vi "Get Error Details (Default).vi"(11 "error":errorcluster) -> (1 "Message":string, 2 "Stack Trace":string, 3 "Type":string)   [LabVIEW 2013, in "JUnit Conversion.lvlib"]
uses:
  JUnit Conversion.lvlib
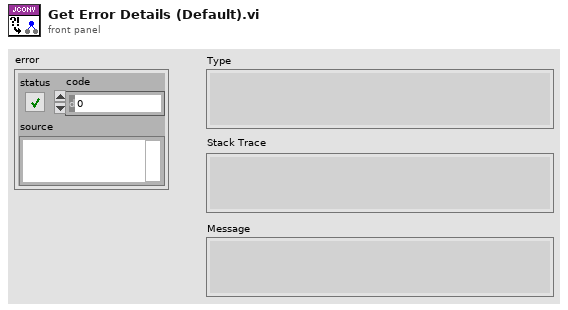
[diagram p1: front panel]
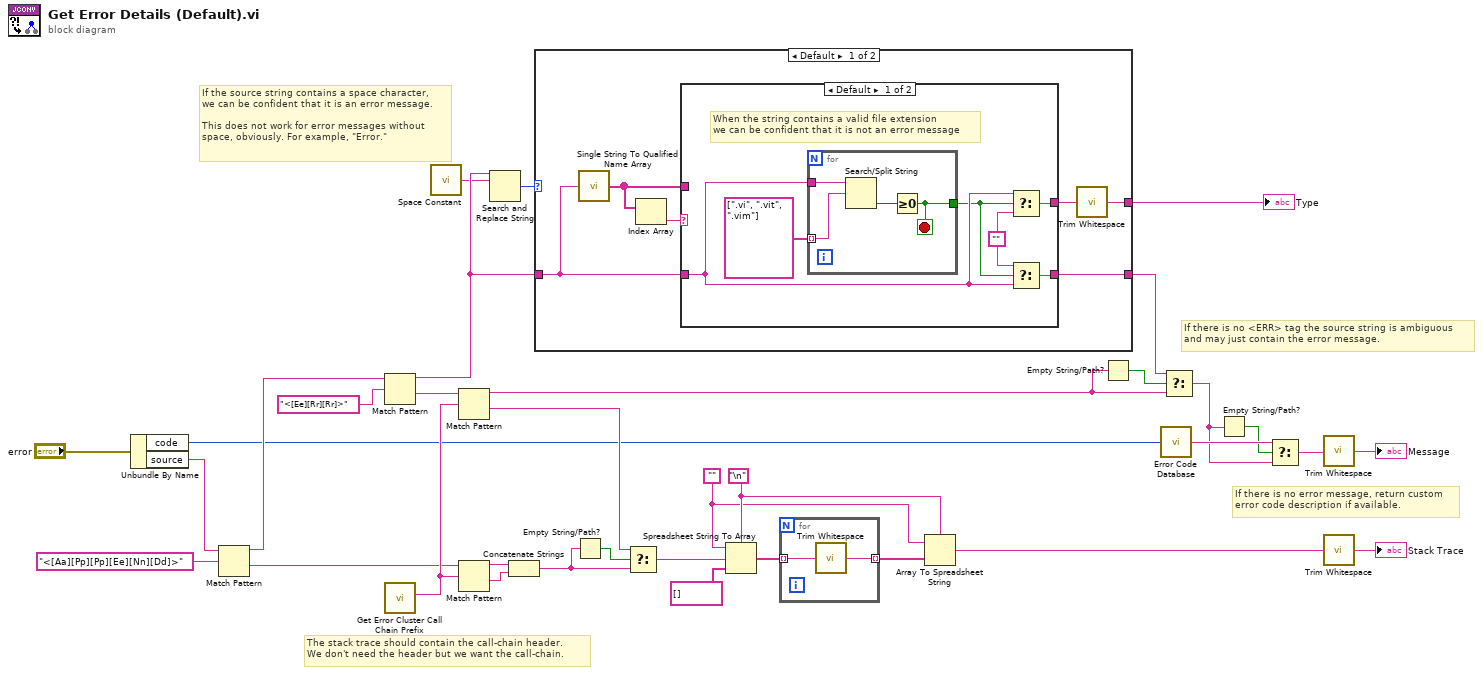
[diagram p0: block diagram]
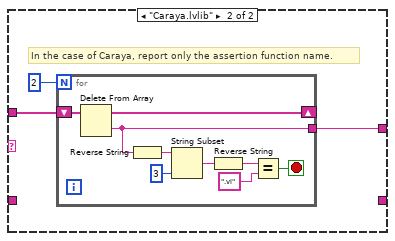
[diagram p2: hidden frame]
diagram:
  w27 = ""
  w28 = "\n"
  # "If the source string contains a space character,\nwe can be confident that it is an error message.\n\nThis does not work for error messages without\nspace, obviously. For example, \"Error.\""
  # "If there is no error message, return custom\nerror code description if available."
  # "The stack trace should contain the call-chain header.\nWe don't need the header but we want the call-chain."
  # "If there is no <ERR> tag the source string is ambiguous\nand may just contain the error message."
  n1 = Unbundle By Name("error") -> ("code"=w11:i32, "source"=w15:string)
  n2 = Match Pattern(string=w15, regular expression="<[Aa][Pp][Pp][Ee][Nn][Dd]>") -> (before substring=w14:string, after substring=w13:string)  [unwired: 1 in, 2 out]
  n3 = Match Pattern(string=w14, regular expression="<[Ee][Rr][Rr]>") -> (before substring=w4:string, after substring=w18:string)  [unwired: 1 in, 2 out]
  n4 = call "Get Error Cluster Call Chain Prefix.vi"() -> ("Call Chain Prefix"=w20:string)  [unwired: 11 in]
  n5 = call <vilib>:"Space Constant.vi"() -> ("String"=w3:string)
  n6 = Match Pattern(string=w18, regular expression=w20) -> (before substring=w5:string, after substring=w19:string)  [unwired: 1 in, 2 out]
  n7 = Match Pattern(string=w13, regular expression=w20) -> (before substring=w23:string, after substring=w22:string)  [unwired: 1 in, 2 out]
  n8 = Search and Replace String(input string=w4, search string=w3) -> (number of replacements=w2:i32)  [unwired: 6 in, 3 out]
  n9 = Concatenate Strings(w23, w22) -> (w21:string)
  n10 = case shown="Default" w2 {
    tunnel: [w36 _] -> w12
    tunnel: w4 -> [w38 w63]
    tunnel: [w35 w63] -> w1
    frame Default {
      n11 = call <vilib>:"Single String To Qualified Name Array.vi"("Fully Qualified String"=w38) -> ("Fully Qualified Array"=w40:string[])
      n12 = Index Array(array=w40) -> (element=w39:string)  [unwired: 1 in]
      n13 = case shown="Default" w39 {
        tunnel: w40 -> [_ w53]
        tunnel: [w45 w51] -> w37
        tunnel: w38 -> [w42 _]
        tunnel: [w44 _] -> w35
        frame Default {
          w43 = ""
          # "When the string contains a valid file extension\nwe can be confident that it is not an error message"
          n14 = for {
            tunnel: w42 -> [w50]
            tunnel: string[] [".vi", ".vit", ".vim"] -> [w49] mode=indexing
            tunnel: [w47] -> w41
            stop <- w47 stop-if-true
            n15 = Search/Split String(string=w50, search string/char (-)=w49) -> (offset of match=w48:i32)  [unwired: 1 in, 2 out]
            n16 = Greater Or Equal To 0?(x=w48) -> (x >= 0?=w47:bool)
          }
          n17 = Select(t=w42, s=w41, f=w43) -> (s? t:f=w45:string)
          n18 = Select(t=w43, s=w41, f=w42) -> (s? t:f=w44:string)
        }
        frame "Caraya.lvlib" {
          # "In the case of Caraya, report only the assertion function name."
          n19 = for {
            N: 2 -> [_]
            shift-right: [w61] -> _
            shift-left: w53 -> [w62]
            tunnel: [w54] -> w51
            stop <- w55 stop-if-true
            n20 = Delete From Array(array=w62) -> (deleted portion=w54:string, array with subset deleted=w61:string[])  [unwired: 2 in]
            n21 = Reverse String(1:w54) -> (0:w60:string)
            n22 = String Subset(string=w60, length (rest)=3 ("length (rest)")) -> (substring=w58:string)  [unwired: 1 in]
            n23 = Reverse String(1:w58) -> (0:w57:string)
            n24 = Equal?(x=w57, y=".vi") -> (x = y?=w55:bool)
          }
        }
      }
      n25 = call <vilib>:"Trim Whitespace.vi"("string"=w37) -> ("trimmed string"=w36:string)  [unwired: 1 in]
    }
    frame 1 {
    }
  }
  "Type" <- w12
  n26 = Empty String/Path?(string/path=w21) -> (empty?=w25:bool)
  n27 = Select(t=w19, s=w25, f=w21) -> (s? t:f=w24:string)
  n28 = Spreadsheet String To Array(delimiter (Tab)=w28, format string=w27, spreadsheet string=w24, array type (2D Dbl)=string[] []) -> (array=w31:string[])
  n29 = for {
    tunnel: [w65] -> w30 mode=indexing
    tunnel: w31 -> [w64] mode=indexing
    n30 = call <vilib>:"Trim Whitespace.vi"("string"=w64) -> ("trimmed string"=w65:string)  [unwired: 1 in]
  }
  n31 = Array To Spreadsheet String(delimiter (Tab)=w28, array=w30, 3:w27) -> (spreadsheet string=w29:string)
  n32 = Empty String/Path?(string/path=w5) -> (empty?=w6:bool)
  n33 = call <vilib>:"Error Code Database.vi"("Error Code"=w11) -> ("Error Text"=w10:string)
  n34 = Select(t=w1, s=w6, f=w5) -> (s? t:f=w8:string)
  n35 = Empty String/Path?(string/path=w8) -> (empty?=w9:bool)
  n36 = Select(t=w10, s=w9, f=w8) -> (s? t:f=w7:string)
  n37 = call <vilib>:"Trim Whitespace.vi"("string"=w7) -> ("trimmed string"=→"Message":string)  [unwired: 1 in]
  n38 = call <vilib>:"Trim Whitespace.vi"("string"=w29) -> ("trimmed string"=→"Stack Trace":string)  [unwired: 1 in]
